vi "MEMR-Open IPC.vi"() -> (8 "IPC":T1)   [LabVIEW 2020]
uses:
  Typedefs/MEMR-IPC.ctl
  Typedefs/MEMR-Params.ctl
  Typedefs/MEMR-Probe.ctl
  Typedefs/MEMR-Elicitor.ctl
  Human Studies/SFM Frontend/LV Source/Typedefs/HSTS-Transducer.ctl
  Typedefs/MEMR-Sequence.ctl
  Typedefs/MEMR-Analysis.ctl
  Typedefs/MEMR-Timing.ctl
  CFTS Main Panel SubVIs/CFTS-Experiment State.ctl
  Typedefs/MEMR-Sequence Step.ctl
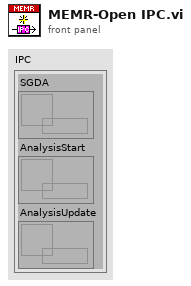
[diagram p1: front panel]
types:
  T1 = typedef "MEMR-IPC.ctl" = cluster{"SGDA":refnum<queue>, "AnalysisStart":refnum<queue>, "AnalysisUpdate":refnum<queue>}
  T2 = typedef "MEMR-Sequence Step.ctl" = cluster{"seq":i32, "rep":i32}
  T3 = typedef "MEMR-Params.ctl" = cluster{"Probe":T4, "Elicitor":T5, "Sequence":T7, "Analysis":T8, "Repeats":i32, "Timing":T9, "Save raw":bool, "Fs (Hz)":dbl}
  T4 = typedef "MEMR-Probe.ctl" = cluster{"Ear":enum16{"Right", "Left"}, "Stimulus":enum16{"Click", "Chirp"}, "Duration (us)":dbl, "Level":dbl}
  T5 = typedef "MEMR-Elicitor.ctl" = cluster{"Duration (ms)":dbl, "Ramp (ms)":dbl, "Transducer":T6}
  T6 = typedef "HSTS-Transducer.ctl" = enum16{"Insert", "TDH-39", "HD300", "ER-10X"}
  T7 = typedef "MEMR-Sequence.ctl" = cluster{"Start":dbl, "Stop":dbl, "Step":dbl}
  T8 = typedef "MEMR-Analysis.ctl" = cluster{"T(ms) re peak":dbl, "Fmin (Hz)":dbl, "Fmax (Hz)":dbl, "Window":enum16{"None", "Hanning", "Hamming"}, "Gain (dB)":dbl, "Resol (Hz)":dbl}
  T9 = typedef "MEMR-Timing.ctl" = cluster{"Click1-Noise (ms)":dbl, "Noise-Click2 (ms)":dbl, "ISI (ms)":dbl}
  T10 = typedef "CFTS-Experiment State.ctl" = cluster{"Experimenter":string, "Number":u32, "Right":string, "Left":string, "Data Folder":path, "State File":path, "Version Info":string, "End Exposure Time":dbl, "Exposure Duration":string, "Run #":cluster{"CAP":i16, "ABR":i16, "DP":i16, "VsEP":i16, "MeasSeq":i16, "SubSeq":i16, "SFOAE":i16}}
  T11 = cluster{"queue out":refnum<queue>, "queue out":refnum<queue>, "queue out":refnum<queue>}
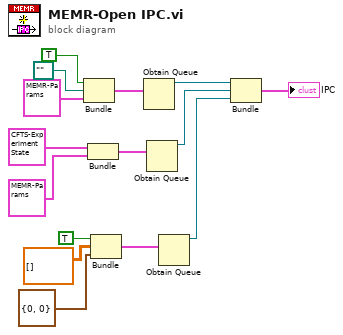
[diagram p0: block diagram]
diagram:
  n1 = Bundle(TRUE, path "", "Params"=T3 {"Probe"={"Ear"=enum."Right", "Stimulus"=enum."Click", "Duration (us)"=0.0, "Level"=0.0}, "Elicitor"={"Duration (ms)"=0.0, "Ramp (ms)"=0.0, "Transducer"=enum."Insert"}, "Sequence"={"Start"=0.0, "Stop"=0.0, "Step"=0.0}, "Analysis"={"T(ms) re peak"=0.0, "Fmin (Hz)"=0.0, "Fmax (Hz)"=0.0, "Window"=enum."None", "Gain (dB)"=0.0, "Resol (Hz)"=0.0}, "Repeats"=0, "Timing"={"Click1-Noise (ms)"=0.0, "Noise-Click2 (ms)"=0.0, "ISI (ms)"=0.0}, "Save raw"=FALSE, "Fs (Hz)"=0.0}) -> (w14:cluster{bool, path, "Params":T3})  [unwired: 1 in]
  n2 = Bundle("Expt State"=T10 {"Experimenter"="", "Number"=0, "Right"="", "Left"="", "Data Folder"=path "", "State File"=path "", "Version Info"="", "End Exposure Time"=0.0, "Exposure Duration"="", "Run #"={"CAP"=0, "ABR"=0, "DP"=0, "VsEP"=0, "MeasSeq"=0, "SubSeq"=0, "SFOAE"=0}}, "Params"=T3 {"Probe"={"Ear"=enum."Right", "Stimulus"=enum."Click", "Duration (us)"=0.0, "Level"=0.0}, "Elicitor"={"Duration (ms)"=0.0, "Ramp (ms)"=0.0, "Transducer"=enum."Insert"}, "Sequence"={"Start"=0.0, "Stop"=0.0, "Step"=0.0}, "Analysis"={"T(ms) re peak"=0.0, "Fmin (Hz)"=0.0, "Fmax (Hz)"=0.0, "Window"=enum."None", "Gain (dB)"=0.0, "Resol (Hz)"=0.0}, "Repeats"=0, "Timing"={"Click1-Noise (ms)"=0.0, "Noise-Click2 (ms)"=0.0, "ISI (ms)"=0.0}, "Save raw"=FALSE, "Fs (Hz)"=0.0}) -> (w8:cluster{"Expt State":T10, "Params":T3})  [unwired: 1 in]
  n3 = Bundle(TRUE, dbl[][] [], "Step Out"=T2 {"seq"=0, "rep"=0}) -> (w11:cluster{bool, dbl[][], "Step Out":T2})  [unwired: 1 in]
  n4 = Obtain Queue(element data type=w14) -> (queue out=w7:refnum<queue>)  [unwired: 4 in, 2 out]
  n5 = Obtain Queue(element data type=w8) -> (queue out=w6:refnum<queue>)  [unwired: 4 in, 2 out]
  n6 = Obtain Queue(element data type=w11) -> (queue out=w5:refnum<queue>)  [unwired: 4 in, 2 out]
  n7 = Bundle("queue out"=w7, "queue out"=w6, "queue out"=w5) -> (→"IPC":T11)  [unwired: 1 in]
